vi "Encode IR Parameters.vi"(8 "ADD Parameters (in)":string, 9 "Scanner Settings In":T2={"Scan1"=1, "Scan2"=1, "Scan3"=1, "Scan4"=1, "Scan5"=1, "Scan6"=1, "Scan7"=1, "Scan8"=1, "Scan9"=1, "Scan10"=1, "Scan11"=1, "Scan12"=1, "Scan13"=1, "Scan14"=1, "Scan15"=1, "Scan16"=1} {"Scan16" scale=0.0..2.0; "Scan15" scale=0.0..2.0; "Scan14" scale=0.0..2.0; "Scan13" scale=0.0..2.0; "Scan12" scale=0.0..2.0; "Scan11" scale=0.0..2.0; "Scan10" scale=0.0..2.0; "Scan9" scale=0.0..2.0; "Scan8" scale=0.0..2.0; "Scan7" scale=0.0..2.0; "Scan6" scale=0.0..2.0; "Scan5" scale=0.0..2.0; "Scan4" scale=0.0..2.0; "Scan3" min=0 max=2 scale=0.0..2.0; "Scan2" min=0 max=2 scale=0.0..2.0; "Scan1" min=0 max=2 scale=0.0..2.0}, 10 "Internal Scanner Exists?":bool, 11 "IR Test Parameters In":T1={"Voltage (10~3000V)"=1000, "High Limit(0.0, 0.1~50,000 Mohms)"=0.0, "Low Limit(0.1~50,000 Mohms)"=0.1, "Ramp Up Time (0.1~999.9 seconds)"=0.1, "Delay Time (0.5~999.9 seconds)"=0.5, "Ramp Down Time (0.0, 1.0~999.9 seconds)"=0.0, "Charge LO  (0.000~3.500uA)"=0.0, "Auto Charge LO (F: Off)"=FALSE, "Dwell Time (0.5~999.9 seconds, 0 = Constant)"=0.5} {"Dwell Time (0.5~999.9 seconds, 0 = Constant)" format="%.1f"; "Ramp Down Time (0.0, 1.0~999.9 seconds)" format="%.1f"; "Charge LO  (0.000~3.500uA)" format="%.2f"; "Delay Time (0.5~999.9 seconds)" format="%.1f"; "Ramp Up Time (0.1~999.9 seconds)" format="%.1f"; "Low Limit(0.1~50,000 Mohms)" format="%.1f"; "High Limit(0.0, 0.1~50,000 Mohms)" format="%.1f"}) -> (1 "Scanner Settings Out":T2={"Scan1"=1, "Scan2"=1, "Scan3"=1, "Scan4"=1, "Scan5"=1, "Scan6"=1, "Scan7"=1, "Scan8"=1, "Scan9"=1, "Scan10"=1, "Scan11"=1, "Scan12"=1, "Scan13"=1, "Scan14"=1, "Scan15"=1, "Scan16"=1} {"Scan16" scale=0.0..2.0; "Scan15" scale=0.0..2.0; "Scan14" scale=0.0..2.0; "Scan13" scale=0.0..2.0; "Scan12" scale=0.0..2.0; "Scan11" scale=0.0..2.0; "Scan10" scale=0.0..2.0; "Scan9" scale=0.0..2.0; "Scan8" scale=0.0..2.0; "Scan7" scale=0.0..2.0; "Scan6" scale=0.0..2.0; "Scan5" scale=0.0..2.0; "Scan4" scale=0.0..2.0; "Scan3" min=0 max=2 scale=0.0..2.0; "Scan2" min=0 max=2 scale=0.0..2.0; "Scan1" min=0 max=2 scale=0.0..2.0}, 2 "IR Test Parameters Out":T1={"Voltage (10~3000V)"=1000, "High Limit(0.0, 0.1~50,000 Mohms)"=0.0, "Low Limit(0.1~50,000 Mohms)"=0.1, "Ramp Up Time (0.1~999.9 seconds)"=0.1, "Delay Time (0.5~999.9 seconds)"=0.5, "Ramp Down Time (0.0, 1.0~999.9 seconds)"=0.0, "Charge LO  (0.000~3.500uA)"=0.0, "Auto Charge LO (F: Off)"=FALSE, "Dwell Time (0.5~999.9 seconds, 0 = Constant)"=0.5} {"Dwell Time (0.5~999.9 seconds, 0 = Constant)" format="%.1f"; "Ramp Down Time (0.0, 1.0~999.9 seconds)" format="%.1f"; "Charge LO  (0.000~3.500uA)" format="%.2f"; "Delay Time (0.5~999.9 seconds)" format="%.1f"; "Ramp Up Time (0.1~999.9 seconds)" format="%.1f"; "Low Limit(0.1~50,000 Mohms)" format="%.1f"; "High Limit(0.0, 0.1~50,000 Mohms)" format="%.1f"}, 3 "ADD command":string)   [LabVIEW 2016, in "eec EST 300.lvlib"]
uses:
  <instrlib>/eec EST 300/eec EST 300.lvlib
  <instrlib>/eec EST 300/Public/Configure/Steps/Low Level/IR Test Parameters.ctl
  <instrlib>/eec EST 300/Public/Configure/Steps/Low Level/Scanner Settings.ctl
panel:
  # "On\nOff"
  # "On\nOff"
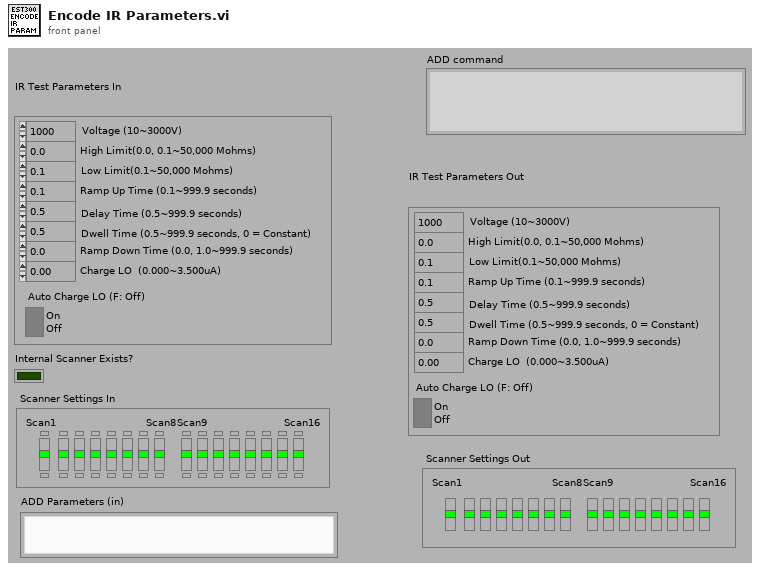
[diagram p1: front panel]
types:
  T1 = typedef "eec EST 300.lvlib/IR Test Parameters.ctl" = cluster{"Voltage (10~3000V)":i64, "High Limit(0.0, 0.1~50,000 Mohms)":dbl, "Low Limit(0.1~50,000 Mohms)":dbl, "Ramp Up Time (0.1~999.9 seconds)":dbl, "Delay Time (0.5~999.9 seconds)":dbl, "Ramp Down Time (0.0, 1.0~999.9 seconds)":dbl, "Charge LO  (0.000~3.500uA)":dbl, "Auto Charge LO (F: Off)":bool, "Dwell Time (0.5~999.9 seconds, 0 = Constant)":dbl}
  T2 = typedef "eec EST 300.lvlib/Scanner Settings.ctl" = cluster{"Scan1":i32, "Scan2":i32, "Scan3":i32, "Scan4":i32, "Scan5":i32, "Scan6":i32, "Scan7":i32, "Scan8":i32, "Scan9":i32, "Scan10":i32, "Scan11":i32, "Scan12":i32, "Scan13":i32, "Scan14":i32, "Scan15":i32, "Scan16":i32}
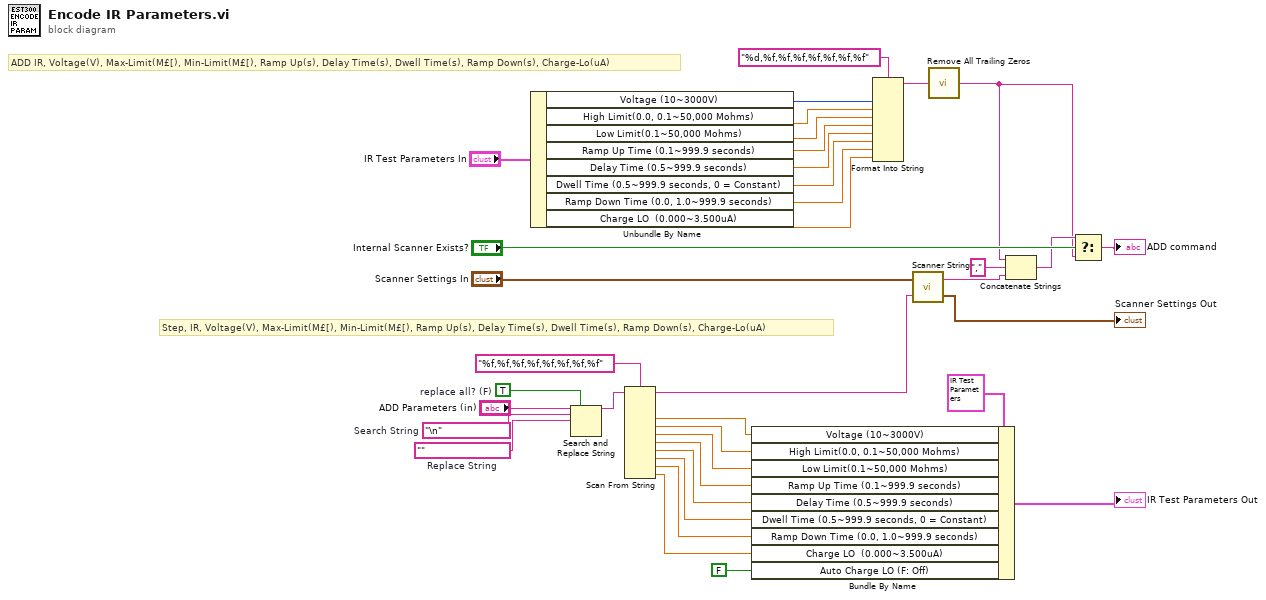
[diagram p0: block diagram]
diagram:
  w24 = TRUE  # replace all? (F)
  w25 = ""  # Replace String
  w26 = "\n"  # Search String
  # "Step, IR, Voltage(V), Max-Limit(M£[), Min-Limit(M£[), Ramp Up(s), Delay Time(s), Dwell Time(s), Ramp Down(s), Charge-Lo(uA)"
  # "ADD IR, Voltage(V), Max-Limit(M£[), Min-Limit(M£[), Ramp Up(s), Delay Time(s), Dwell Time(s), Ramp Down(s), Charge-Lo(uA)"
  n1 = Unbundle By Name("IR Test Parameters In") -> ("Voltage (10~3000V)"=w37:i64, "High Limit(0.0, 0.1~50,000 Mohms)"=w36:dbl, "Low Limit(0.1~50,000 Mohms)"=w35:dbl, "Ramp Up Time (0.1~999.9 seconds)"=w34:dbl, "Delay Time (0.5~999.9 seconds)"=w21:dbl, "Dwell Time (0.5~999.9 seconds, 0 = Constant)"=w33:dbl, "Ramp Down Time (0.0, 1.0~999.9 seconds)"=w32:dbl, "Charge LO  (0.000~3.500uA)"=w31:dbl)
  n2 = Search and Replace String(replace all?=w24, input string="ADD Parameters (in)", search string=w26, replace string=w25) -> (result string=w22:string)  [unwired: 4 in, 3 out]
  n3 = Scan From String(format string="%f,%f,%f,%f,%f,%f,%f,%f" ("Format String"), input string=w22) -> (remaining string=w14:string, output 1=w1:dbl, output 2=w2:dbl, output 3=w8:dbl, output 4=w7:dbl, output 5=w6:dbl, output 6=w5:dbl, output 7=w4:dbl, output 8=w3:dbl)  [unwired: 10 in, 2 out]
  n4 = Bundle By Name(cluster=T1 {"Voltage (10~3000V)"=1000, "High Limit(0.0, 0.1~50,000 Mohms)"=0.0, "Low Limit(0.1~50,000 Mohms)"=0.1, "Ramp Up Time (0.1~999.9 seconds)"=0.1, "Delay Time (0.5~999.9 seconds)"=0.5, "Ramp Down Time (0.0, 1.0~999.9 seconds)"=0.0, "Charge LO  (0.000~3.500uA)"=0.0, "Auto Charge LO (F: Off)"=FALSE, "Dwell Time (0.5~999.9 seconds, 0 = Constant)"=0.5} ("IR Test Parameters Out 2"), "Voltage (10~3000V)"=w1, "High Limit(0.0, 0.1~50,000 Mohms)"=w2, "Low Limit(0.1~50,000 Mohms)"=w8, "Ramp Up Time (0.1~999.9 seconds)"=w7, "Delay Time (0.5~999.9 seconds)"=w6, "Dwell Time (0.5~999.9 seconds, 0 = Constant)"=w5, "Ramp Down Time (0.0, 1.0~999.9 seconds)"=w4, "Charge LO  (0.000~3.500uA)"=w3, "Auto Charge LO (F: Off)"=FALSE) -> (→"IR Test Parameters Out":T1)
  n5 = Format Into String(format string="%d,%f,%f,%f,%f,%f,%f,%f" ("Format String"), w37, w36, w35, w34, w21, w33, w32, w31) -> (resulting string=w12:string)  [unwired: 2 in, 1 out]
  n6 = call <instrlib>:"Scanner String.vi"("Scanner String (in)"=w14, "Scanner Settings in"="Scanner Settings In") -> ("Scanner Settings out"=→"Scanner Settings Out":T2, "Scanner String (out)"=w18:string)
  n7 = call <instrlib>:"Remove All Trailing Zeros.vi"("String in"=w12) -> ("String out"=w11:string)
  n8 = Concatenate Strings(w11, "," ("Substring"), w18) -> (w27:string)
  n9 = Select(t=w27, s="Internal Scanner Exists?", f=w11) -> (s? t:f=→"ADD command":string)
